vi "Add Compact Array Items.vi"(7 "File Refnum":T6, 8 "error in":errorcluster, 9 "Count":u8, 10 "Index":i32, 11 "ODs in":T1[](array[typedef]) {"SubNumber" format="%x"; "AccessType" items=["", "ro", "wo", "rw", "const", "rwr", "rww"]; "DataType" items=[""=0, "BOOLEAN"=1, "INTEGER8"=2, "INTEGER16"=3, "INTEGER32"=4, "UNSIGNED8"=5, "UNSIGNED16"=6, "UNSIGNED32"=7, "REAL32"=8, "VISIBLE_STRING"=9, "OCTET_STRING"=10, "UNICODE_STRING"=11, "TIME_OF_DAY"=12, "TIME_DIFFERENCE"=13, "DOMAIN"=15, "INTEGER24"=16, "REAL64"=17, "INTEGER40"=18, "INTEGER48"=19, "INTEGER56"=20, "INTEGER64"=21, "UNSIGNED24"=22, "UNSIGNED40"=24, "UNSIGNED48"=25, "UNSIGNED56"=26, "UNSIGNED64"=27]; "ObjectType" items=[""=10, "NULL"=0, "DOMAIN"=2, "DEFTYPE"=5, "DEFSTRUCT"=6, "VAR"=7, "ARRAY"=8, "RECORD"=9]; "sub-index" format="%x"; "index" format="%x"}) -> (0 "error out":errorcluster, 2 "Next Index":i32, 3 "ODs out":T1[](array[typedef]) {"SubNumber" format="%x"; "AccessType" items=["", "ro", "wo", "rw", "const", "rwr", "rww"]; "DataType" items=[""=0, "BOOLEAN"=1, "INTEGER8"=2, "INTEGER16"=3, "INTEGER32"=4, "UNSIGNED8"=5, "UNSIGNED16"=6, "UNSIGNED32"=7, "REAL32"=8, "VISIBLE_STRING"=9, "OCTET_STRING"=10, "UNICODE_STRING"=11, "TIME_OF_DAY"=12, "TIME_DIFFERENCE"=13, "DOMAIN"=15, "INTEGER24"=16, "REAL64"=17, "INTEGER40"=18, "INTEGER48"=19, "INTEGER56"=20, "INTEGER64"=21, "UNSIGNED24"=22, "UNSIGNED40"=24, "UNSIGNED48"=25, "UNSIGNED56"=26, "UNSIGNED64"=27]; "ObjectType" items=[""=10, "NULL"=0, "DOMAIN"=2, "DEFTYPE"=5, "DEFSTRUCT"=6, "VAR"=7, "ARRAY"=8, "RECORD"=9]; "sub-index" format="%x"; "index" format="%x"})   [LabVIEW 2021, in "CANOpen Addon System Explorer.lvlib"]
uses:
  CANOpen Addon System Explorer.lvlib
  <vilib>/Utility/config.llb/Config Data RefNum.ctl
  control/OD Entry.ctl
  control/Object Type.ctl
  control/Data Type.ctl
  control/Access Type.ctl
  control/OD Cateory.ctl
  <vilib>/Utility/config.llb/Read Key (String).vi
  <vilib>/Utility/config.llb/NI_LVConfig.lvlib
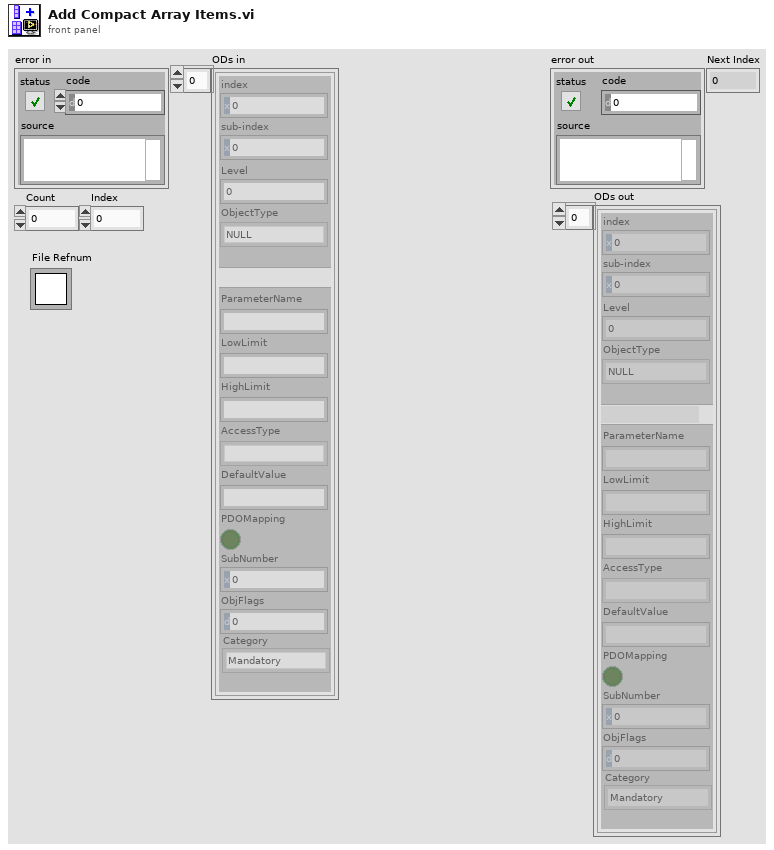
[diagram p1: front panel]
types:
  T1 = typedef "CANOpen Addon System Explorer.lvlib/OD Entry.ctl" = cluster{"index":u16, "sub-index":u8, "Level":u8, "ObjectType":T2, "DataType":T3, "ParameterName":string, "LowLimit":string, "HighLimit":string, "AccessType":T4, "DefaultValue":string, "PDOMapping":bool, "SubNumber":u8, "ObjFlags":u32, "Category":T5}
  T2 = typedef "CANOpen Addon System Explorer.lvlib/Object Type.ctl" = u16
  T3 = typedef "CANOpen Addon System Explorer.lvlib/Data Type.ctl" = u16
  T4 = typedef "CANOpen Addon System Explorer.lvlib/Access Type.ctl" = u16
  T5 = typedef "CANOpen Addon System Explorer.lvlib/OD Cateory.ctl" = enum16{"Mandatory", "Optional", "Manufacturer", ""}
  T6 = typedef "NI_LVConfig.lvlib/Config Data RefNum.ctl" = refnum<k1>
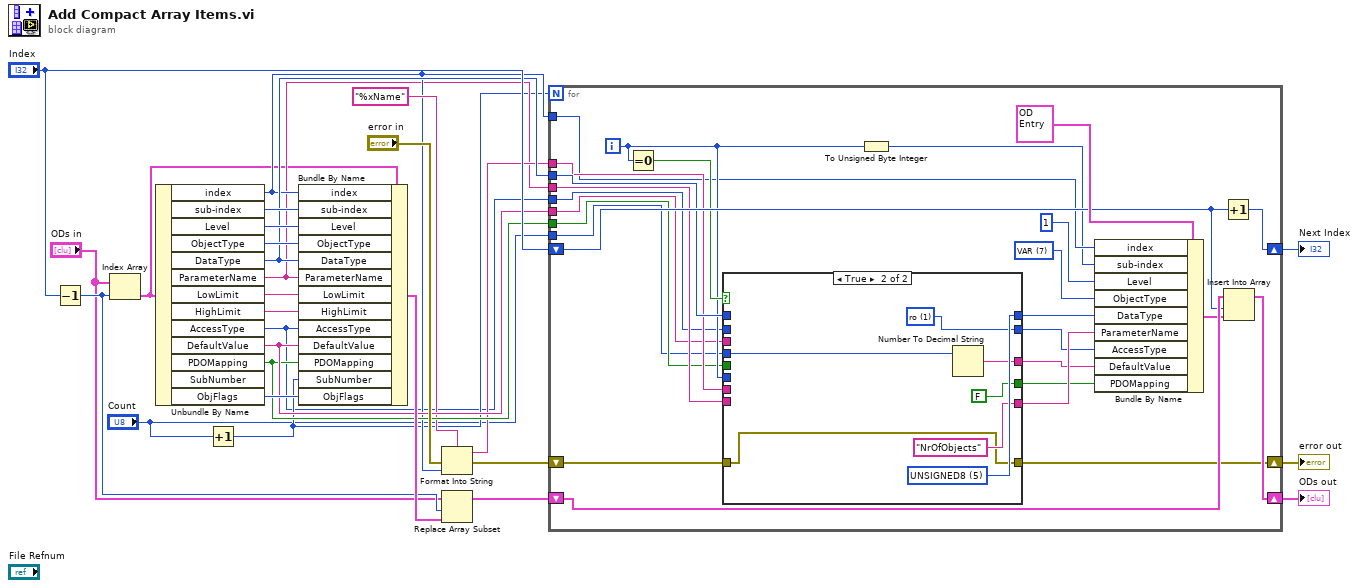
[diagram p0: block diagram]
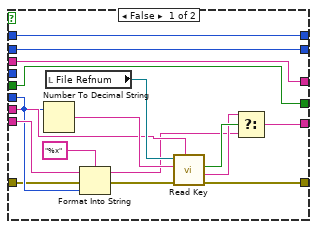
[diagram p2: hidden frame]
diagram:
  n1 = Decrement(x="Index") -> (x-1=w14:i32)
  n2 = Index Array(array="ODs in", index=w14) -> (element=w4:T1)
  n3 = Unbundle By Name(w4) -> ("index"=w9:u16, "sub-index"=w22:u8, "Level"=w21:u8, "ObjectType"=w20:T2, "DataType"=w13:T3, "ParameterName"=w6:string, "LowLimit"=w19:string, "HighLimit"=w18:string, "AccessType"=w1:T4, "DefaultValue"=w12:string, "PDOMapping"=w11:bool, "ObjFlags"=w17:u32)  [unwired: 1 out]
  n4 = Increment(x="Count") -> (x+1=w3:u8)
  n5 = Bundle By Name(cluster=w4, "index"=w9, "sub-index"=w22, "Level"=w21, "ObjectType"=w20, "DataType"=w13, "ParameterName"=w6, "LowLimit"=w19, "HighLimit"=w18, "AccessType"=w1, "DefaultValue"=w12, "PDOMapping"=w11, "SubNumber"=w3, "ObjFlags"=w17) -> (w16:T1)
  n6 = Format Into String(format string="%xName", error in="error in", w9) -> (resulting string=w7:string, error out=w8:errorcluster)  [unwired: 1 in]
  n7 = Replace Array Subset(array="ODs in", new element=w16, index=w14) -> (w15:T1[])
  n8 = for {
    N: w3 -> [_]
    shift-right: [w52] -> w24
    shift-left: w15 -> [w53]
    shift-right: [w48] -> w23
    shift-left: "Index" -> [w49]
    tunnel: w9 -> [w38]
    tunnel: w13 -> [w44]
    tunnel: "Count" -> [w29]
    tunnel: w1 -> [w34]
    tunnel: w12 -> [w36]
    tunnel: w11 -> [w32]
    shift-right: [w30] -> w26
    shift-left: w8 -> [w31]
    tunnel: w7 -> [w41]
    tunnel: w6 -> [w40]
    i -> [w42]
    w46 = T2 7 items=[""=10, "NULL"=0, "DOMAIN"=2, "DEFTYPE"=5, "DEFSTRUCT"=6, "VAR"=7, "ARRAY"=8, "RECORD"=9] ("ObjectType")
    n9 = Equal To 0?(x=w42) -> (x = 0?=w45:bool)
    n10 = case shown="True" w45 {
      tunnel: [w70 w77] -> w43
      tunnel: w44 -> [w70 _]
      tunnel: [w64 "NrOfObjects" ("LowLimit")] -> w39
      tunnel: w42 -> [w61 _]
      tunnel: w41 -> [w67 _]
      tunnel: w40 -> [w63 _]
      tunnel: w29 -> [_ w72]
      tunnel: [w59 w75] -> w37
      tunnel: w36 -> [w59 _]
      tunnel: [w54 w71] -> w35
      tunnel: w34 -> [w54 _]
      tunnel: [w58 FALSE ("t")] -> w33
      tunnel: w32 -> [w58 _]
      tunnel: w31 -> [w57 w73]
      tunnel: [w55 w73] -> w30
      frame False {
        n11 = Number To Decimal String(number=w61) -> (decimal integer string=w68:string)  [unwired: 1 in]
        n12 = local read "File Refnum"() -> (w69:T6)
        n13 = Format Into String(format string="%x", initial string=w63, error in=w57, w61) -> (resulting string=w60:string, error out=w56:errorcluster)
        n14 = call-poly <vilib>:"Read Key.vi"("section"=w67, "error in (no error)"=w56, "key"=w68, "refnum"=w69) -> ("error out"=w55:errorcluster, "value"=w65:string, "found?"=w66:bool)  [unwired: 4 in, 1 out]
        n15 = Select(t=w65, s=w66, f=w60) -> (s? t:f=w64:string)
      }
      frame True {
        w71 = T4 1 items=["", "ro", "wo", "rw", "const", "rwr", "rww"] ("AccessType")
        w77 = T3 5 items=[""=0, "BOOLEAN"=1, "INTEGER8"=2, "INTEGER16"=3, "INTEGER32"=4, "UNSIGNED8"=5, "UNSIGNED16"=6, "UNSIGNED32"=7, "REAL32"=8, "VISIBLE_STRING"=9, "OCTET_STRING"=10, "UNICODE_STRING"=11, "TIME_OF_DAY"=12, "TIME_DIFFERENCE"=13, "DOMAIN"=15, "INTEGER24"=16, "REAL64"=17, "INTEGER40"=18, "INTEGER48"=19, "INTEGER56"=20, "INTEGER64"=21, "UNSIGNED24"=22, "UNSIGNED40"=24, "UNSIGNED48"=25, "UNSIGNED56"=26, "UNSIGNED64"=27] ("DataType")
        n16 = Number To Decimal String(number=w72) -> (decimal integer string=w75:string)  [unwired: 1 in]
      }
    }
    n17 = To Unsigned Byte Integer(number=w42) -> (unsigned 8bit integer=w28:u8)
    n18 = Bundle By Name(cluster=T1 {"index"=0, "sub-index"=0, "Level"=0, "ObjectType"=10, "DataType"=0, "ParameterName"="", "LowLimit"="", "HighLimit"="", "AccessType"=0, "DefaultValue"="", "PDOMapping"=FALSE, "SubNumber"=0, "ObjFlags"=0, "Category"=enum."Mandatory"} ("element"), "index"=w38, "sub-index"=w28, "Level"=u8 1, "ObjectType"=w46, "DataType"=w43, "ParameterName"=w39, "AccessType"=w35, "DefaultValue"=w37, "PDOMapping"=w33) -> (w51:T1)
    n19 = Increment(x=w49) -> (x+1=w48:i32)
    n20 = Insert Into Array(array=w53, index=w49, new element=w51) -> (w52:T1[])
  }
  "error out" <- w26
  "ODs out" <- w24
  "Next Index" <- w23
